vi "Dense.vi"(1 "b":dbl[][](array[numeric]), 2 "A":dbl[][](array[numeric]), 3 "w":dbl[][](array[numeric])) -> (0 "Z":dbl[][](array[numeric]))   [LabVIEW 2020]
uses:
  <vilib>/Analysis/baseanly.llb/Real A x B.vi
  <vilib>/Analysis/Matrix/Numeric/Conversions/Array To Matrix - RA2.vi
  <vilib>/Analysis/Matrix/Numeric/Conversions/Matrix To Array - RM.vi
  <vilib>/Analysis/NI_AALBase.lvlib
  <vilib>/Analysis/Matrix/NI_Matrix.lvlib
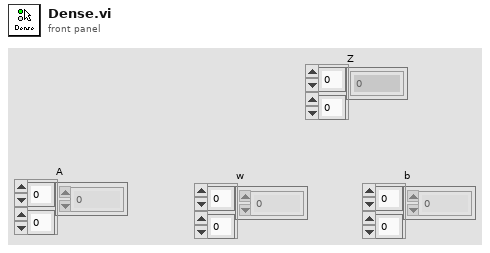
[diagram p1: front panel]
types:
  T1 = typedef "NI_Matrix.lvlib/RealMatrix.ctl" = dbl[][]
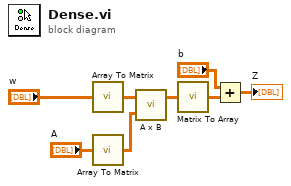
[diagram p0: block diagram]
diagram:
  n1 = call-poly <vilib>:"Array To Matrix.vi"("Real 2D Array"="w") -> ("Real Matrix"=w5:T1)
  n2 = call-poly <vilib>:"Array To Matrix.vi"("Real 2D Array"="A") -> ("Real Matrix"=w6:T1)
  n3 = call-poly <vilib>:"A x B.vi"("B"=w6, "A"=w5) -> ("A x B"=w4:T1)  [unwired: 1 out]
  n4 = call-poly <vilib>:"Matrix To Array.vi"("Real Matrix"=w4) -> ("Real 2D Array"=w3:dbl[][])
  n5 = Add(x="b", y=w3) -> (x+y=→"Z":dbl[][])
